vi "CAN debug.vi"() -> ()   [LabVIEW 2019]
uses:
  <vilib>/RioEmbeddedCAN/RioEmbeddedCAN.llb/CANFrameControl.ctl
panel:
  out "output array":u8[](array[numeric])
  out "error out":errorcluster
  in  "debug":bool
  out "appended array 2":u8[][](array[numeric])
  out "appended array":u32[](array[numeric]) format="%.0x"
  in  "stop":bool
  out "timestamp":timestamp
  in  "baud rate":u32=500000
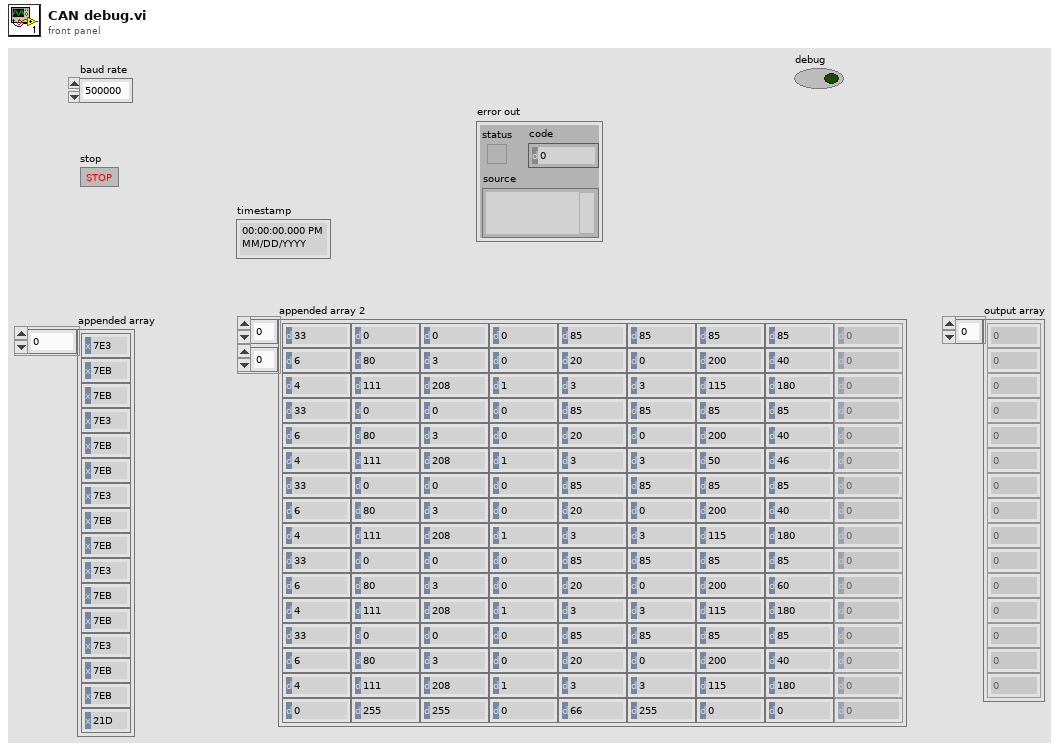
[diagram p1: front panel]
types:
  T1 = typedef "CANFrameControl.ctl" = cluster{"identifier":u32, "extended?":bool, "type":u8, "payload":u8[]}
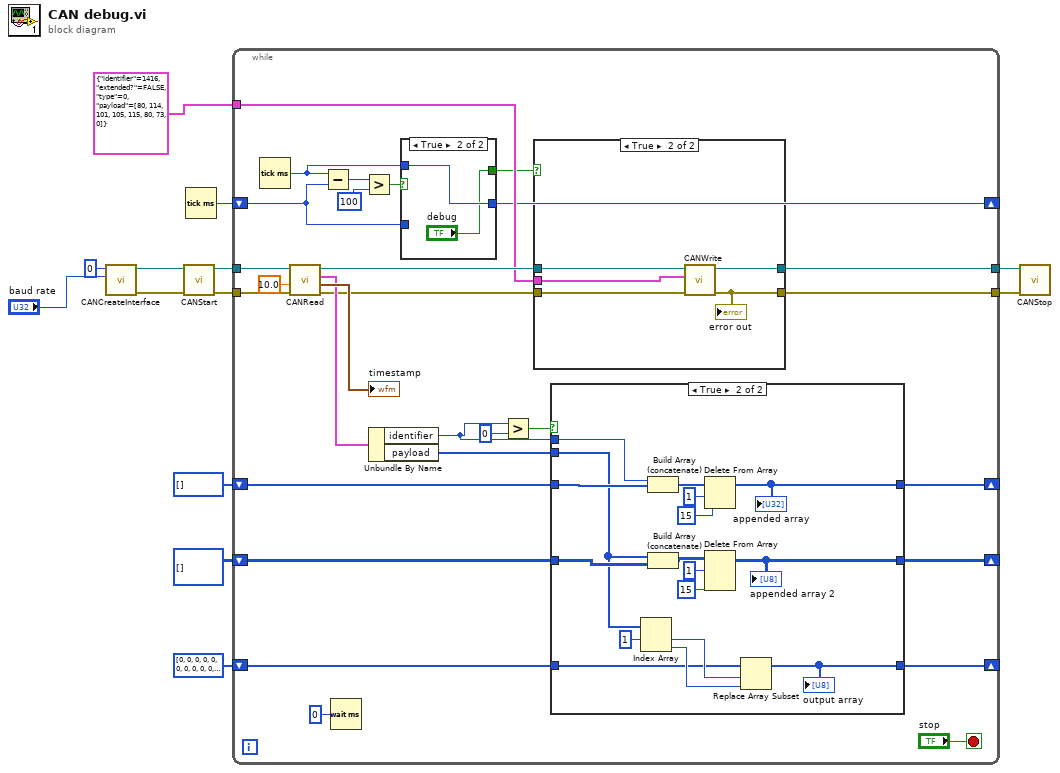
[diagram p0: block diagram]
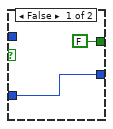
[diagram p2: hidden frame]
diagram:
  n1 = call <vilib>:"CANCreateInterface.vi"("baud rate (125000 bps)"="baud rate", "interface index"=u32 0) -> ("error out"=w10:errorcluster, "interface object out"=w11:refnum<k20>)  [unwired: 8 in]
  n2 = call <vilib>:"CANStart.vi"("error in (no error)"=w10, "interface object in"=w11) -> ("error out"=w7:errorcluster, "interface object out"=w9:refnum<k20>)  [unwired: 8 in]
  n3 = Tick Count (ms)() -> (millisecond timer value=w2:u32)
  n4 = while {
    tunnel: w9 -> [w42]
    tunnel: [w25] -> w8
    tunnel: w7 -> [w40]
    tunnel: [w24] -> w6
    shift-right: [w31] -> _
    shift-left: u8[][] [] -> [w29]
    shift-right: [w32] -> _
    shift-left: u32[] [] -> [w30]
    tunnel: T1 {"identifier"=1416, "extended?"=FALSE, "type"=0, "payload"=[80, 114, 101, 105, 115, 80, 73, 0]} ("CAN frame") -> [w23]
    shift-right: [w19] -> _
    shift-left: w2 -> [w20]
    shift-right: [w15] -> _
    shift-left: u8[] [0, 0, 0, 0, 0, 0, 0, 0, 0, 0, 0, 0, 0, 0] -> [w14]
    stop <- "stop" stop-if-true
    n5 = Tick Count (ms)() -> (millisecond timer value=w18:u32)
    n6 = call <vilib>:"CANRead.vi"("error in (no error)"=w40, "timeout (0 s)"=10.0 ("timeout"), "interface object in"=w42) -> ("error out"=w26:errorcluster, "timestamp"=→"timestamp":timestamp, "CAN frame"=w37:T1, "interface object out"=w27:refnum<k20>)  [unwired: 5 in]
    n7 = Subtract(x=w18, y=w20) -> (x-y=w16:u32)
    n8 = Wait (ms)(milliseconds to wait=u32 0) -> ()  [unwired: 1 out]
    n9 = Greater?(x=w16, y=u32 100) -> (0:w21:bool)
    n10 = Unbundle By Name(w37) -> ("identifier"=w33:u32, "payload"=w34:u8[])
    n11 = case shown="True" w21 {
      tunnel: w20 -> [w44 _]
      tunnel: [w44 w46] -> w19
      tunnel: w18 -> [_ w46]
      tunnel: [FALSE ("debug") "debug"] -> w17
      frame False {
      }
      frame True {
      }
    }
    n12 = Greater?(x=w33, y=u32 0) -> (0:w35:bool)
    n13 = case shown="True" w17 {
      tunnel: w27 -> [w48 w53]
      tunnel: w26 -> [w47 w52]
      tunnel: [w48 w51] -> w25
      tunnel: [w47 w50] -> w24
      tunnel: w23 -> [_ w49]
      frame False {
      }
      frame True {
        n14 = call <vilib>:"CANWrite.vi"("error in (no error)"=w52, "CAN frame"=w49, "interface object in"=w53) -> ("error out"=w50:errorcluster, "interface object out"=w51:refnum<k20>)  [unwired: 7 in]
        "error out" <- w50
      }
    }
    n15 = case shown="True" w35 {
      tunnel: w34 -> [_ w62]
      tunnel: w33 -> [_ w73]
      tunnel: [w56 w69] -> w32
      tunnel: [w55 w63] -> w31
      tunnel: w30 -> [w56 w71]
      tunnel: w29 -> [w55 w70]
      tunnel: [w54 w58] -> w15
      tunnel: w14 -> [w54 w57]
      frame False {
      }
      frame True {
        n16 = Index Array(array=w62, index #1=1 ("index")) -> (element #1=w60:u8, element #2=w59:u8)  [unwired: 1 in]
        n17 = Build Array (concatenate)(w73, w71) -> (w72:u32[])
        n18 = Build Array (concatenate)(w62, w70) -> (w64:u8[][])
        n19 = Delete From Array(array=w72, length=1, index=15) -> (array with subset deleted=w69:u32[])  [unwired: 1 out]
        "appended array" <- w69
        n20 = Delete From Array(array=w64, length=1, index (row)=15 ("index")) -> (array with subset deleted=w63:u8[][])  [unwired: 1 in, 1 out]
        "appended array 2" <- w63
        n21 = Replace Array Subset(array=w57, new element=w59, index=w60) -> (w58:u8[])
        "output array" <- w58
      }
    }
  }
  n22 = call <vilib>:"CANStop.vi"("error in (no error)"=w6, "interface object in"=w8) -> ()  [unwired: 8 in, 2 out]
